vi "MoveSinglePIMotor_Mercury.vi"(0 "System no.":i32=1 min=1 step=1, 1 "Axes to move":string[](array[string]), 3 "Move":dbl[](array[numeric]) format="%.6f", 5 "error in":errorcluster, 11 "Move":bool, 12 "Stop refnum":refnum<vi>) -> (15 "Position":dbl[](array[numeric]) format="%.6f", 19 "error out":errorcluster)   [LabVIEW 2013]
doc: "This VI is runs in a loop until the stop button is pressed, the stop reference is TRUE or an error occures. It lets the operator set the velocity, move the connected axes to relative, absolute or to the home position, and reads the current position continuosly. The diagram shows how to combine the driver and support VIs for these tasks. Use the Help?Show Context Help menu sequence in the LabVIEW environment to display the Context Help window with the VI and control/indicator descriptions.\nRun \" XXXX_Configuration_Setup.vi\" (with XXXX being the PI product number of your system) prior to running this VI. \n\nValid for: C-843, C-843.PM, C-865, C-866, Mercury"
uses:
  C:/Users/Public/PI/GCSMergedLabVIEW/Low Level/General command.llb/Global2 (Array).vi
panel:
  in  "stop":bool
  out "Conn. Axes":string[](array[string])
  # "Command move:"
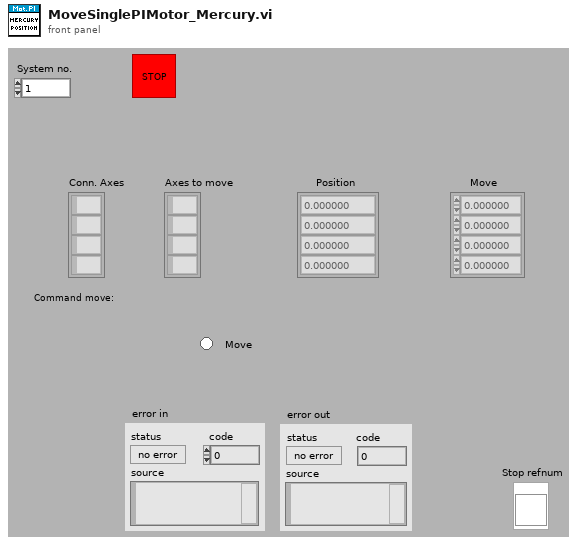
[diagram p1: front panel]
types:
  T1 = typedef "Controller names.ctl" = enum16{"None", "Analog", "C-702", "C-413", "C-843", "C-843.PM", "C-844", "C-848", "C-865", "C-866", "C-867", "C-877", "C-880", "C-884", "C-885", "C-891", "E-516", "E-517", "E-518", "E-709", "E-710", "E-712", "E-725", "E-727", "E-753", "E-754", "E-755", "E-761", "E-816", "E-861", "E-870", "E-871", "E-873", "F-206", "HydraPollux", "M-840", "M-850", "M-8X0", "Mercury", "Mercury_GCS"}
  T2 = cluster{"Conn. axes":string[], "Controller name":T1}[]
  T3 = cluster{"Conn. axes":string[], "Controller name":T1}
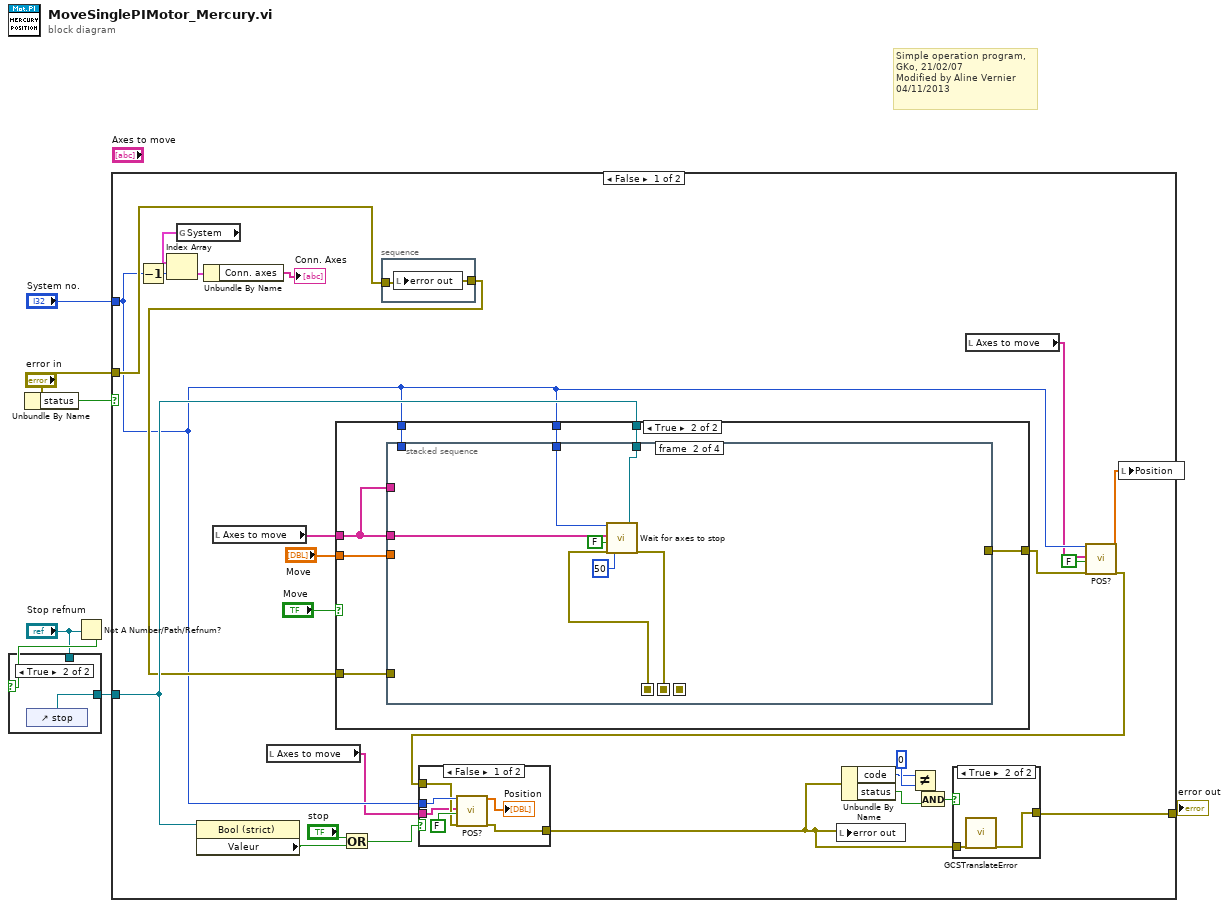
[diagram p0: block diagram]
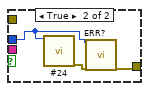
[diagram p4: hidden frame]
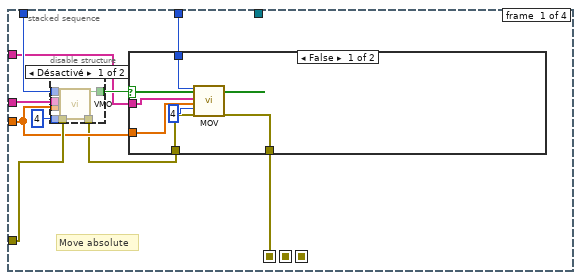
[diagram p6: hidden frame]
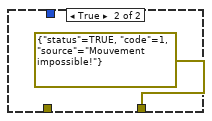
[diagram p8: hidden frame]
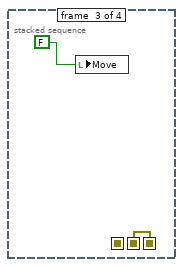
[diagram p9: hidden frame]
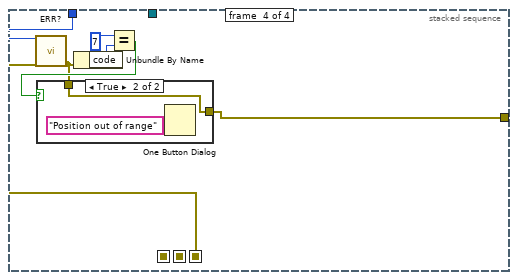
[diagram p10: hidden frame]
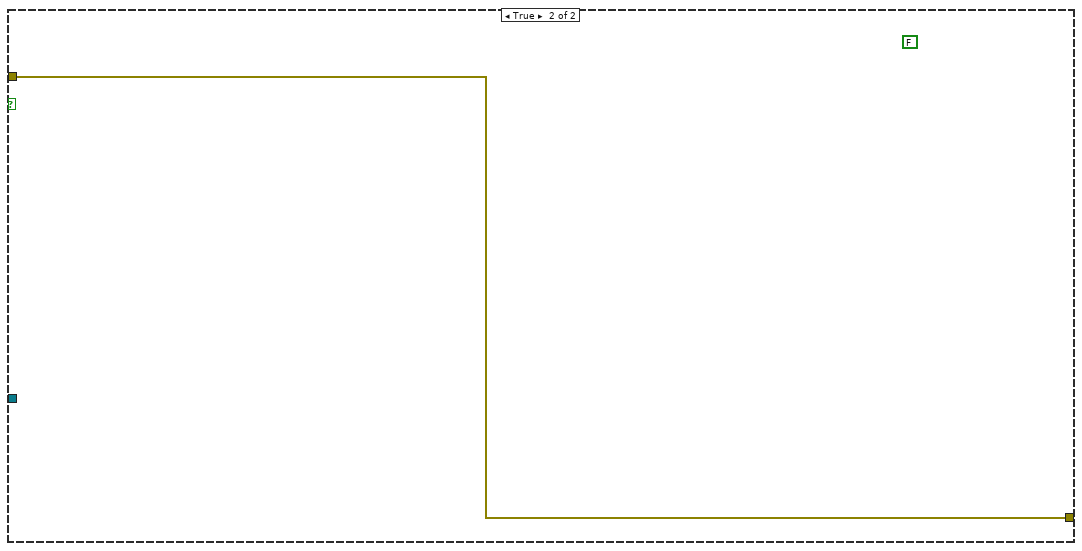
[diagram p12: hidden frame]
diagram:
  # "Simple operation program,\nGKo, 21/02/07\nModified by Aline Vernier\n04/11/2013"
  n1 = Unbundle By Name("error in") -> ("status"=w6:bool)
  n2 = Not A Number/Path/Refnum?(number/path/refnum="Stop refnum") -> (NaN/Path/Refnum?=w3:bool)
  n3 = case shown="True" w3 {
    tunnel: [w8 w9] -> w2
    tunnel: "Stop refnum" -> [w8 _]
    frame False {
    }
    frame True {
      n4 = control-ref of="stop"() -> (w9:refnum<vi>)
    }
  }
  n5 = case shown="False" w6 {
    tunnel: [w36 w101] -> w5
    tunnel: "error in" -> [w35 w101]
    tunnel: "System no." -> [w15 _]
    tunnel: w2 -> [w34 _]
    frame False {
      n6 = Decrement(x=w15) -> (x-1=w33:i32)
      n7 = global read "Global2 (Array).vi" "System"() -> (w32:T2)
      n8 = Index Array(array=w32, index=w33) -> (element=w31:T3)
      n9 = property class="Bool (strict)"(reference=w34) -> ("Valeur"=w27:bool)  [unwired: 1 in, 2 out]
      n10 = Unbundle By Name(w31) -> ("Conn. axes"=→"Conn. Axes":string[])
      n11 = local read "Axes to move"() -> (w18:string[])
      n12 = local read "Axes to move"() -> (w10:string[])
      n13 = Or(x="stop", y=w27) -> (x .or. y?=w24:bool)
      n14 = stacked-sequence {
        tunnel: w35 -> [w100]
        tunnel: [w100] -> w30
        frame #0 {
          n15 = local write "error out"(w100) -> ()
        }
      }
      n16 = case shown="True" "Move" {
        tunnel: w15 -> [_ w56]
        tunnel: "Move" -> [_ w55]
        tunnel: w34 -> [_ w54]
        tunnel: w30 -> [w49 w53]
        tunnel: w15 -> [_ w52]
        tunnel: w18 -> [_ w50]
        tunnel: [w49 w51] -> w16
        frame False {
        }
        frame True {
          n17 = stacked-sequence {
            seq-local: [w62 _ _ _] -> [_ w83 _ _]
            seq-local: [_ w82 _ _] -> [_ _ w88 _]
            seq-local: [_ _ w88 _] -> [_ _ _ w91]
            tunnel: w56 -> [w66 w85 _ w94]
            tunnel: w55 -> [w64 _ _ _]
            tunnel: w54 -> [_ w84 _ _]
            tunnel: w53 -> [w65 _ _ _]
            tunnel: w52 -> [w63 _ _ _]
            tunnel: w50 -> [w58 w81 _ _]
            tunnel: [_ _ _ w90] -> w51
            tunnel: w50 -> [w57 _ _ _]
            frame #0 {
              # "Move absolute"
              n18 = disable-structure shown="Désactivé" {
                disable-tunnel: w65 -> [w73 _]
                disable-tunnel: w64 -> [w72 _]
                disable-tunnel: w63 -> [w71 _]
                disable-tunnel: i16 4 ("No.of digits") -> [w70 _]
                disable-tunnel: [w69 _] -> w60
                disable-tunnel: [w68 _] -> w59
                disable-tunnel: w58 -> [w67 _]
                frame Disabled {
                  n19 = call "VMO.vi"("System no."=w71, "Axes to command"=w67, "Position values"=w72, "No.of digits"=w70, "error in"=w73) -> ("Move possible"=w69:bool, "error out"=w68:errorcluster)  [unwired: 13 in]
                }
                frame Enabled {
                }
              }
              n20 = case shown="False" w60 {
                tunnel: w66 -> [w78 _]
                tunnel: w64 -> [w77 _]
                tunnel: w59 -> [w76 _]
                tunnel: [w75 errorcluster {"status"=TRUE, "code"=1, "source"="Mouvement impossible!"} ("error in")] -> w62
                tunnel: w57 -> [w74 _]
                frame False {
                  n21 = call "MOV.vi"("System no."=w78, "Axes to move"=w74, "Position values"=w77, "No.of digits"=i16 4, "error in"=w76) -> ("error out"=w75:errorcluster)  [unwired: 14 in]
                }
                frame True {
                }
              }
            }
            frame #1 {
              n22 = call "Wait for axes to stop.vi"("System no."=w85, "Axes to wait for"=w81, "With status bit polling?"=FALSE, "error in"=w83, "Polling cycle time, ms"=u32 50, "Stop refnum"=w84) -> ("error out"=w82:errorcluster)  [unwired: 12 in, 1 out]
            }
            frame #2 {
              n23 = local write "Move"(FALSE ("Go home")) -> ()
            }
            frame #3 {
              n24 = call "ERR?.vi"("System no."=w94, "error in"=w91) -> ("error out"=w93:errorcluster)  [unwired: 16 in, 1 out]
              n25 = Unbundle By Name(w93) -> ("code"=w92:i32)
              n26 = Equal?(x=7 ("y"), y=w92) -> (x = y?=w95:bool)
              n27 = case shown="True" w95 {
                tunnel: [w97 w98] -> w90
                tunnel: w93 -> [w97 w98]
                frame False {
                }
                frame True {
                  n28 = One Button Dialog(message="Position out of range") -> ()  [unwired: 1 in, 1 out]
                }
              }
            }
          }
        }
      }
      n29 = local read "Axes to move"() -> (w14:string[])
      n30 = call "POS?.vi"("System no."=w15, "Axes to query"=w14, "All axes?"=FALSE, "error in"=w16) -> ("Position"=w11:dbl[], "error out"=w12:errorcluster)  [unwired: 14 in]
      n31 = case shown="False" w24 {
        tunnel: w15 -> [w42 w48]
        tunnel: [w44 w46] -> w19
        tunnel: w12 -> [w41 _]
        tunnel: w10 -> [w40 _]
        frame False {
          n32 = call "POS?.vi"("System no."=w42, "Axes to query"=w40, "All axes?"=FALSE, "error in"=w41) -> ("Position"=→"Position":dbl[], "error out"=w44:errorcluster)  [unwired: 14 in]
        }
        frame True {
          n33 = call "#24.vi"("System no."=w48) -> ("error out"=w47:errorcluster)  [unwired: 18 in]
          n34 = call "ERR?.vi"("System no."=w48, "error in"=w47) -> ("error out"=w46:errorcluster)  [unwired: 16 in, 1 out]
        }
      }
      n35 = local write "error out"(w19) -> ()
      n36 = Unbundle By Name(w19) -> ("code"=w21:i32, "status"=w20:bool)
      n37 = Not Equal?(x=w21, y=0 ("code")) -> (x != y?=w26:bool)
      n38 = And(x=w26, y=w20) -> (x .and. y?=w25:bool)
      n39 = case shown="True" w25 {
        tunnel: [w37 w39] -> w36
        tunnel: w19 -> [w37 w38]
        frame False {
        }
        frame True {
          n40 = call "GCSTranslateError.vi"("error in"=w38) -> ("error out"=w39:errorcluster)  [unwired: 16 in, 2 out]
        }
      }
      n41 = local write "Position"(w11) -> ()
    }
    frame True {
      (unwired) FALSE ("stop")
    }
  }
  "error out" <- w5
